vi "Volt Channels Write.vi"(4 "error in (no error)":errorcluster, 5 "Value":string[](array[string]), 6 "Container State":T2, 7 "Display State In":T1) -> (0 "error out":errorcluster, 3 "Display State Out":T1)   [LabVIEW 2013, in "Sensor X.xctl"]
uses:
  Sensor X.xctl
  <vilib>/_xctls/Container State.ctl
  Sensor X State.ctl
  <vilib>/_xctls/XControlSupport.lvlib
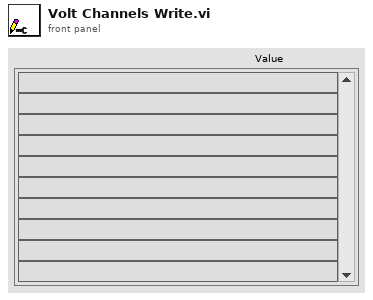
[diagram p1: front panel]
types:
  T1 = typedef "Sensor X.xctl/Sensor X State.ctl" = cluster{"Volt Channels":string[]}
  T2 = typedef "XControlSupport.lvlib/Container State.ctl" = cluster{"Indicator?":bool, "Run Mode?":bool, " Refnum":refnum<vi>}
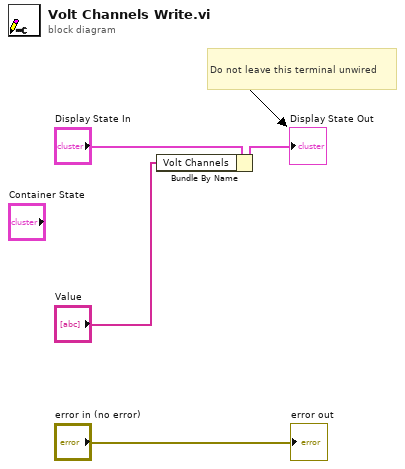
[diagram p0: block diagram]
diagram:
  # "Do not leave this terminal unwired"
  n1 = Bundle By Name(cluster="Display State In", "Volt Channels"="Value") -> (→"Display State Out":T1)
  "error out" <- "error in (no error)"
